vi "load image perspective calibration.vi"(8 "error in (no error)":errorcluster, 11 "Calibration File Path":path) -> (0 "error out":errorcluster, 3 "Refnum out":T1)   [LabVIEW 2020]
uses:
  <vilib>/vision/Image Controls.llb/IMAQ Image.ctl
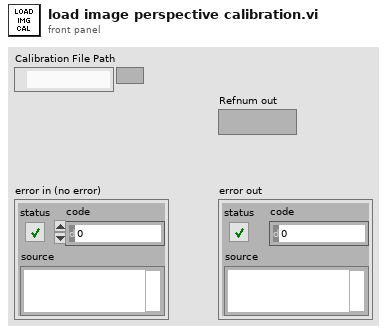
[diagram p1: front panel]
types:
  T1 = typedef "IMAQ Image.ctl" = refnum<image>
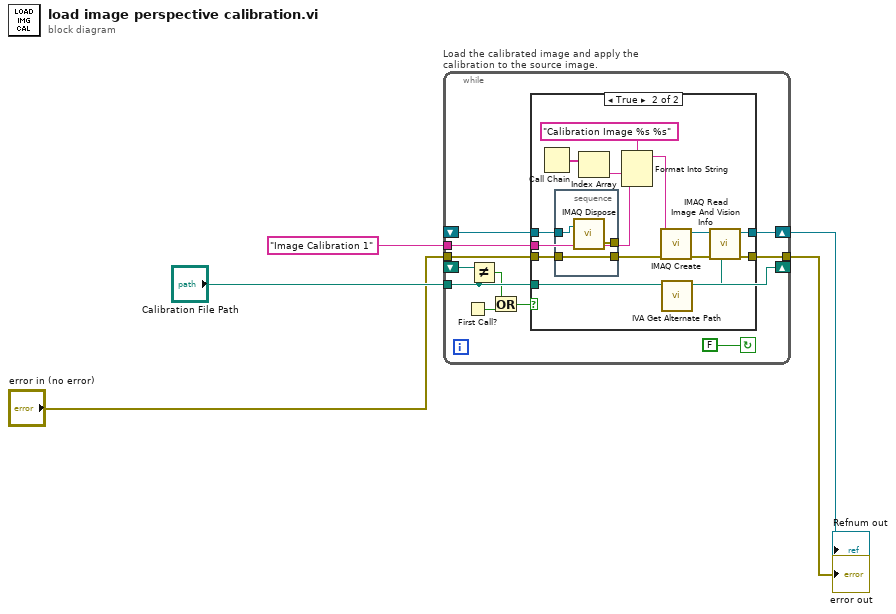
[diagram p0: block diagram]
diagram:
  n1 = while "Load the calibrated image and apply the calibration to the source image." {
    shift-right: [w16] -> w3
    shift-left: _ -> [w15]
    tunnel: [w13] -> w4
    tunnel: "error in (no error)" -> [w12]
    tunnel: "Calibration File Path" -> [w9]
    tunnel: "Image Calibration 1" ("Step Name") -> [w11]
    shift-right: [w9] -> _
    shift-left: _ -> [w10]
    stop <- FALSE continue-if-true
    n2 = First Call?() -> (First Call?: T/F=w8:bool)
    n3 = Not Equal?(x=w10, y=w9) -> (x != y?=w7:bool)
    n4 = Or(x=w7, y=w8) -> (x .or. y?=w6:bool)
    n5 = case shown="True" w6 {
      tunnel: [w18 w30] -> w16
      tunnel: w15 -> [w18 w22]
      tunnel: [w17 w27] -> w13
      tunnel: w12 -> [w17 w23]
      tunnel: w9 -> [_ w20]
      tunnel: w11 -> [_ w24]
      frame False {
      }
      frame True {
        n6 = Call Chain() -> (call chain=w26:string[])
        n7 = stacked-sequence {
          tunnel: w23 -> [w34]
          tunnel: w22 -> [w35]
          tunnel: [w34] -> w21
          tunnel: [w33] -> _
          frame #0 {
            n8 = call "IMAQ Dispose"("Image"=w35) -> ("error out"=w33:errorcluster)  [unwired: 2 in, 3 out]
          }
        }
        n9 = Index Array(array=w26) -> (element=w25:string)  [unwired: 1 in]
        n10 = Format Into String(format string="Calibration Image %s %s" ("Image Name"), w25, w24) -> (resulting string=w32:string)  [unwired: 2 in, 1 out]
        n11 = call "IMAQ Create"("Image Name"=w32, "error in (no error)"=w21) -> ("New Image"=w29:T1, "error out"=w28:errorcluster)  [unwired: 2 in, 1 out]
        n12 = call <vilib>:"IVA Get Alternate Path.vi"("Path In"=w20) -> ("Path Out"=w19:path)  [unwired: 10 out]
        n13 = call "IMAQ Read Image And Vision Info"("File Path"=w19, "error in (no error)"=w28, "Image"=w29) -> ("error out"=w27:errorcluster, "Image Out"=w30:T1)  [unwired: 1 in, 6 out]
      }
    }
  }
  "error out" <- w4
  "Refnum out" <- w3
